vi "testCerebellumNumeric.vi"() -> ()   [LabVIEW 2013]
uses:
  Cerebellum/Cerebellum.lvclass
panel:
  out "PC Right":dbl
  in  "Right Hem Path":path
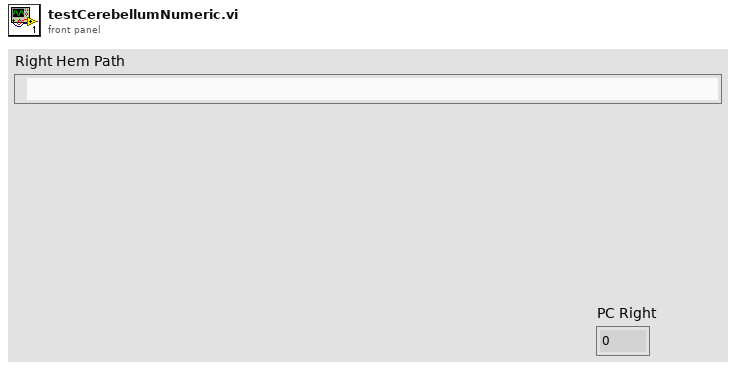
[diagram p1: front panel]
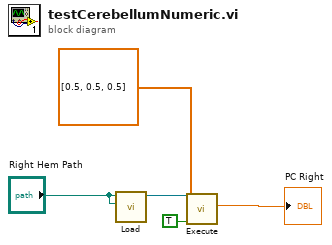
[diagram p0: block diagram]
diagram:
  n1 = call "Load.vi"("Left Hem Path"="Right Hem Path", "Right Hem Path"="Right Hem Path") -> ("Cerebellum out"=w4:refnum<class "Cerebellum.lvclass">)  [unwired: 9 in]
  n2 = call "Execute.vi"("Active?"=TRUE, "Inputs"=dbl[] [0.5, 0.5, 0.5], "Cerebellum in"=w4) -> ("PC Right"=→"PC Right":dbl)  [unwired: 6 in, 2 out]
